vi "GUI_Single Button Pump.vi"() -> ()   [LabVIEW 2011] (continued)
            w1635 = T32[] [enum."Is BLT2 at Atmospheric Pressure?", enum."Is the EC Roughing Manifold at Atmospheric Pressure"] items=["No Action", "Is EC GPM Mode ON?", "Is EC GPM Mode Off?", "Is EC GVM Mode ON?", "Is EC GVM Off?", "Is  EC GPM or GVM Mode ON?", "Is LB GPM Mode ON?", "Is LB GPM Mode Off?", "Is LB GVM Mode ON?", "Is LB GVM Mode Off?", "Is  LB GPM or GVM Mode ON?", "Is M123 Turbo Gate Valve Opened? ", "Is M123 Turbo Gate Valve Closed?", "Is OAP Turbo Gate Valve Opened?", "Is OAP Turbo Gate Valve Closed?", "Is BTLTurbo Gate Valve Opened?", "Is BTL Turbo Gate Valve Closed?", "Is TARGET Turbo Gate Valve 1Opened?", "Is TARGET1 Turbo Gate Valve Closed?", "Is TARGET Turbo Gate Valve 2 Opened?", "Is TAREGT2 Turbo Gate Valve Closed?", "Is BTL2 Turbo Gate Valve Opened?", "Is BTL2 Turbo Gate Valve Closed?", "Is HPD Turbo Gate Valve Opened?", "Is HPD Turbo Gate Valve Closed?", "Is COMP to M123 gate Valve Opened?", "Is COMP to M123 Valve Closed?", "Is HPBD Gate Valve Opened?", "Is HPBD Gate Valve Closed?", "Is M123 to OAP gate valve opened?", "Is M123 to OAP gate valve closed?", "Is OAP to BLT gate valve opened?", "Is OAP to BTL Gate Valve Closed?", "Is BLT to TARGET gate valve opened?", "Is BTL to TARGET Gate Valve Closed?", "Is TARGET to BLT2 gate valve opened?", "Is TARGET to BTL2 Gate Valve Closed?", "Is BLT2 to HPD gate valve opened?", "Is BTL2 to HPD Gate Valve Closed?", "Is COMP at Atmospheric Pressure?", "Is M123 at Atmospheric Pressure?", "Is BeamDump at Atmospheric Pressure?", "Is OAP at Atmospheric Pressure?", "Is BLT at Atmospheric Pressure", "Is TARGET at Atmospheric Pressure?", "Is BLT2 at Atmospheric Pressure?", "Is HPD at Atmospheric Pressure?", "Is the EC Roughing Pump ON?", "Is the EC Roughing Pump OFF?", "Does the EC Roughing Pump have a fault?", "Is the LB Roughing Pump ON?", "Is the LB Roughing Pump Off?", "Does the LB Roughing Pump have a fault?", "Is the EC Backing Pump ON?", "Is the EC Backing Pump OFF?", "Is the LB Backing Pump ON?", "Is the LB Backing Pump OFF?", "Does the EC Backing Pump have a fault?", "Does the LB Backing Pump have a fault?", "Is the EC Backing Pipe at Atmospheric Pressure", "Is the LB Backing Pipe at Atmospheric Pressure", "Is the EC Backing Manifold at Atmospheric Pressure", "s the LB Backing Manifold at Atmospheric Pressure?", "Is the EC Roughing Pipe at Atmospheric Pressure", "Is the LB Roughing Pipe at Atmospheric Pressure?", "Is the EC Roughing Manifold at Atmospheric Pressure", "Is the LB Roughing Manifold at Atmospheric Pressure", "Is LB Backing Manifold Valve Opened?", "Is EC Backing Manifold Valve Opened?", "Is LB Roughing Manifold Valve Opened?", "Is EC Roughing Manifold Valve Opened?", "Is COMP Roughing Valve Opened?", "Is M123 Roughing Valve Opened?", "Is M123 Roughing Valve Closed?", "Is OAP Roughing Valve Opened?", "Is OAP Roughing Valve Closed?", "Is HPBD Roughing Valve Opened?", "Is HPBD Roughing Valve Closed?", "Is BTL Roughing Valve Opened?", "Is BTL Roughing Valve Closed?", "Is TARGET Roughing Valve Opened?", "Is TARGET Roughing Valve Closed?", "Is BTL2 Roughing Valve Opened?", "Is BTL2 Roughing Valve Closed?", "Is HPD Roughing Valve Opened?", "Is HPD Roughing Valve Closed?", "Is COMP Turbo Backing Valve Opened?", "Is M123 Turbo Backing Valve Opened", "Is HPBD Turbo Backing Valve Opened?", "Is OAP Turbo Backing Valve Opened?", "Is BTL Turbo Backing Valve Opened?", "Is TARGET1 Turbo Backing Valve Opened?", "Is TARGET2 Turbo Backing Valve Opened?", "Is BTL2 Turbo Backing Valve Opened?", "Is HPD Turbo Backing Valve Opened?", "Is M123 Backing at MID-VAC?", "Is OAP Backing at MID-VAC?", "Is TARGET1 Backing at MID-VAC?", "Is TARGET2 Backing at MID-VAC?", "Is BTL Backing at MID-VAC?", "Is BTL2 Backing at MID-VAC?", "Is HPD Backing at MID-VAC?", "Is M123 Turbo in Normal Operation", "Is COMP Turbo in Normal Operation", "Is OAP Turbo in Normal Operation", "Is BTL Turbo in Normal Operation", "Is TARGET1 Turbo in Normal Operation", "Is TARGET2 Turbo in Normal Operation", "Is BTL2 Turbo in Normal Operation", "Is HPD Turbo in Normal Operation", "Is M123 at MID-VAC?", "Is OAP at MID-VAC?", "Is COMP at MID-VAC?", "Is BTL at MID-VAC?", "Is TARGET at MID-VAC?", "Is BTL2 at MID-VAC?", "Is HPD at MID-VAC?"]
          }
          frame "HPD" {
            w1636 = T32[] [enum."Is HPD at Atmospheric Pressure?", enum."Is the EC Roughing Manifold at Atmospheric Pressure"] items=["No Action", "Is EC GPM Mode ON?", "Is EC GPM Mode Off?", "Is EC GVM Mode ON?", "Is EC GVM Off?", "Is  EC GPM or GVM Mode ON?", "Is LB GPM Mode ON?", "Is LB GPM Mode Off?", "Is LB GVM Mode ON?", "Is LB GVM Mode Off?", "Is  LB GPM or GVM Mode ON?", "Is M123 Turbo Gate Valve Opened? ", "Is M123 Turbo Gate Valve Closed?", "Is OAP Turbo Gate Valve Opened?", "Is OAP Turbo Gate Valve Closed?", "Is BTLTurbo Gate Valve Opened?", "Is BTL Turbo Gate Valve Closed?", "Is TARGET Turbo Gate Valve 1Opened?", "Is TARGET1 Turbo Gate Valve Closed?", "Is TARGET Turbo Gate Valve 2 Opened?", "Is TAREGT2 Turbo Gate Valve Closed?", "Is BTL2 Turbo Gate Valve Opened?", "Is BTL2 Turbo Gate Valve Closed?", "Is HPD Turbo Gate Valve Opened?", "Is HPD Turbo Gate Valve Closed?", "Is COMP to M123 gate Valve Opened?", "Is COMP to M123 Valve Closed?", "Is HPBD Gate Valve Opened?", "Is HPBD Gate Valve Closed?", "Is M123 to OAP gate valve opened?", "Is M123 to OAP gate valve closed?", "Is OAP to BLT gate valve opened?", "Is OAP to BTL Gate Valve Closed?", "Is BLT to TARGET gate valve opened?", "Is BTL to TARGET Gate Valve Closed?", "Is TARGET to BLT2 gate valve opened?", "Is TARGET to BTL2 Gate Valve Closed?", "Is BLT2 to HPD gate valve opened?", "Is BTL2 to HPD Gate Valve Closed?", "Is COMP at Atmospheric Pressure?", "Is M123 at Atmospheric Pressure?", "Is BeamDump at Atmospheric Pressure?", "Is OAP at Atmospheric Pressure?", "Is BLT at Atmospheric Pressure", "Is TARGET at Atmospheric Pressure?", "Is BLT2 at Atmospheric Pressure?", "Is HPD at Atmospheric Pressure?", "Is the EC Roughing Pump ON?", "Is the EC Roughing Pump OFF?", "Does the EC Roughing Pump have a fault?", "Is the LB Roughing Pump ON?", "Is the LB Roughing Pump Off?", "Does the LB Roughing Pump have a fault?", "Is the EC Backing Pump ON?", "Is the EC Backing Pump OFF?", "Is the LB Backing Pump ON?", "Is the LB Backing Pump OFF?", "Does the EC Backing Pump have a fault?", "Does the LB Backing Pump have a fault?", "Is the EC Backing Pipe at Atmospheric Pressure", "Is the LB Backing Pipe at Atmospheric Pressure", "Is the EC Backing Manifold at Atmospheric Pressure", "s the LB Backing Manifold at Atmospheric Pressure?", "Is the EC Roughing Pipe at Atmospheric Pressure", "Is the LB Roughing Pipe at Atmospheric Pressure?", "Is the EC Roughing Manifold at Atmospheric Pressure", "Is the LB Roughing Manifold at Atmospheric Pressure", "Is LB Backing Manifold Valve Opened?", "Is EC Backing Manifold Valve Opened?", "Is LB Roughing Manifold Valve Opened?", "Is EC Roughing Manifold Valve Opened?", "Is COMP Roughing Valve Opened?", "Is M123 Roughing Valve Opened?", "Is M123 Roughing Valve Closed?", "Is OAP Roughing Valve Opened?", "Is OAP Roughing Valve Closed?", "Is HPBD Roughing Valve Opened?", "Is HPBD Roughing Valve Closed?", "Is BTL Roughing Valve Opened?", "Is BTL Roughing Valve Closed?", "Is TARGET Roughing Valve Opened?", "Is TARGET Roughing Valve Closed?", "Is BTL2 Roughing Valve Opened?", "Is BTL2 Roughing Valve Closed?", "Is HPD Roughing Valve Opened?", "Is HPD Roughing Valve Closed?", "Is COMP Turbo Backing Valve Opened?", "Is M123 Turbo Backing Valve Opened", "Is HPBD Turbo Backing Valve Opened?", "Is OAP Turbo Backing Valve Opened?", "Is BTL Turbo Backing Valve Opened?", "Is TARGET1 Turbo Backing Valve Opened?", "Is TARGET2 Turbo Backing Valve Opened?", "Is BTL2 Turbo Backing Valve Opened?", "Is HPD Turbo Backing Valve Opened?", "Is M123 Backing at MID-VAC?", "Is OAP Backing at MID-VAC?", "Is TARGET1 Backing at MID-VAC?", "Is TARGET2 Backing at MID-VAC?", "Is BTL Backing at MID-VAC?", "Is BTL2 Backing at MID-VAC?", "Is HPD Backing at MID-VAC?", "Is M123 Turbo in Normal Operation", "Is COMP Turbo in Normal Operation", "Is OAP Turbo in Normal Operation", "Is BTL Turbo in Normal Operation", "Is TARGET1 Turbo in Normal Operation", "Is TARGET2 Turbo in Normal Operation", "Is BTL2 Turbo in Normal Operation", "Is HPD Turbo in Normal Operation", "Is M123 at MID-VAC?", "Is OAP at MID-VAC?", "Is COMP at MID-VAC?", "Is BTL at MID-VAC?", "Is TARGET at MID-VAC?", "Is BTL2 at MID-VAC?", "Is HPD at MID-VAC?"]
          }
        }
        n626 = call "GetAction.vi"("Check Condition"=w1606, "Query Array"=w1609, "input cluster"=w1600, "error in (no error)"=w1610) -> ("Status Array Out"=w1608:string[], "Generate Event?"=w1595:bool, "error out"=w1607:errorcluster)  [unwired: 6 in, 3 out]
        n627 = call "Generate User Event.vi"("Add(t)/Remove(f) Event"=w1595, "error in (no error)"=w1607, "User Event in"=w1612, "Status Array In"=w1608, "Error Codes"=w1606) -> ("error out"=w1611:errorcluster)  [unwired: 5 in, 1 out]
        n628 = case shown="\"M123\"" w1596 {
          tunnel: [w1615 "M123 chamber and the Roughing Manifold do not match in Pressure.\nPress Continue to Wait for 30 Seconds\nPress Exit to Quit" ("message") "HPBD Chamber and Roughing Manifold do not have matching Pressure.\nStop and Exit.(Restart the Pump down after all turbo valves have been manually closed)" ("message") "OAP Chamber and Roughing Manifold do not have matching Pressure.\nStop and Exit.(Restart the Pump down after all turbo valves have been manually closed)" ("message") "BTL Chamber and Roughing Manifold do not have matching Pressure.\nStop and Exit.(Restart the Pump down after all turbo valves have been manually closed)" ("message") "TARGET Chamber and Roughing Manifold do not have matching Pressure.\nStop and Exit.(Restart the Pump down after all turbo valves have been manually closed)" ("message") "BTL2 Chamber and Roughing Manifold do not have matching Pressure.\nStop and Exit.(Restart the Pump down after all turbo valves have been manually closed)" ("message") "HPD Chamber and Roughing Manifold do not have matching Pressure.\nStop and Exit.(Restart the Pump down after all turbo valves have been manually closed)" ("message")] -> w1602
          tunnel: [w1615 "Main: Roughing Valve Precheck>>M123" "Main: Roughing Valve Precheck>>HPBD" "Main: Roughing Valve Precheck>>OAP" "Main: Roughing Valve Precheck>>BTL" "Main: Roughing Valve Precheck>>TARGET" "Main: Roughing Valve Precheck>>BTL2" "Main: Roughing Valve Precheck>>HPD"] -> w1593
          frame "False", Default {
            w1615 = ""
          }
          frame "M123" {
          }
          frame "HPBD" {
          }
          frame "OAP" {
          }
          frame "BTL" {
          }
          frame "TARGET" {
          }
          frame "BTL2" {
          }
          frame "HPD" {
          }
        }
        n629 = call "MID-VAC Timer.vi"("Action"=timerAction_typdef."Timer Running") -> ("TO"=w1604:bool)  [unwired: 10 in]
        n630 = And(x=w1595, y=w1604) -> (x .and. y?=w1603:bool)
        n631 = Unbundle By Name(w1600) -> ("VI Refnum"=w1598:refnum<vi>)
        n632 = control-ref of="User Input Panel"() -> (w1599:refnum<vi>)
        n633 = call "Gen Next State based on user input.vi"("Next State IN"="", "Generate Event?"=w1595, "Idle State"=w1593, "Continue To Wait State"=w1593, "VI Refnum"=w1598, "SubPanel in"=w1599) -> ("Next State Out"=w1594:string)  [unwired: 5 in]
        n634 = call "Generate TO event.vi"("Boolean"=w1603, "message"=w1602, "User Event in"=w1601) -> ()  [unwired: 9 in]
        n635 = call <vilib>:"Add State(s) to Queue__jki_lib_state_machine.vi"("State(s) in Front (\"\")"=w1594, "State(s) in (\"\")"=w1614) -> ("States Out"=w1613:string)  [unwired: 13 in]
      }
      frame "Main: Open Roughing Valve" {
        # "Open Backing Valves on both systems"
        n636 = Unbundle By Name(w1641) -> ("TCPConnection.Command TCP Connection LB"=w1649:refnum<k5>)
        n637 = Unbundle By Name(w1641) -> ("TCPConnection.Command TCP Connection EC"=w1647:refnum<k5>)
        n638 = case shown="\"BTL2\"" w1639 {
          tunnel: [_ w1654 w1655 w1656 _ w1657 w1658 w1659 w1660] -> w1651
          frame "False", Default {
          }
          frame "M123" {
            w1654 = T33[] [enum."Open M123 Roughing Valve"] items=["No Action", "Set GPM Mode LB", "EXIT GPM Mode LB", "Set GPM Mode EC", "EXIT GPM Mode EC", "Set GVM mode LB", "Set GVM Mode EC", "Open LB Backing Valve", "Open EC Backing Valve", "Open EC Roughing Valve", "Open LB Roughing Valve", "Open M123 Roughing Valve", "Close M123 Roughing Valve", "Open Compressor Roughing Valve", "Close Compressor Roughing Valve", "Open BeamDump Roughing Valve", "Close BeamDump Roughing Valve", "Open OAP Roughing Valve", "Close OAP Roughing Valve", "Open BTL Roughing Valve", "Close BTL Roughing Valve", "Open Target Roughing Valve", "Close Target Roughing Valve", "Open BTL2 Roughing Valve", "Close BTL2 Roughing Valve", "Open HPD Roughing Valve", "Close HPD Roughing Valve", "LB Start Roughing Pump ", "EC Start Roughing Pump", "Open COMP Turbo Backing Valve", "Open M123 Turbo Backing Valve", "Open OAP Turbo Backing Valve", "Open HPBD Turbo Backing Valve", "Open BLT Turbo Backing Valve", "Open TARGET1 Turbo Backing Valve", "Open TARGET2 Turbo Backing Valve", "Open BLT2 Turbo Backing Valve", "Open HPD Turbo Backing Valve", "LB Start Turbo Backing Pump", "EC Start Turbo Backing Pump", "Start COMP Turbo Pump", "Start M123 Turbo Pump", "Start OAP Turbo Pump", "Start BTL Turbo Pump", "Start TARGET1 Turbo Pump", "Start TARGET2 Turbo Pump", "Start BTL2 Turbo Pump", "Start HPD Turbo Pump", "Open COMP Turbo Gate Valve", "Open M123 Turbo Gate Valve", "Open OAP Turbo Gate Valve", "Open BTL Turbo Gate Valve", "Open TARGET1 Turbo Gate Valve", "Open TARGET2 Turbo Gate Valve", "Open BTL2 Turbo Gate Valve", "Open HPD Turbo Gate Valve"]
          }
          frame "HPBD" {
            w1655 = T33[] [enum."Open BeamDump Roughing Valve"] items=["No Action", "Set GPM Mode LB", "EXIT GPM Mode LB", "Set GPM Mode EC", "EXIT GPM Mode EC", "Set GVM mode LB", "Set GVM Mode EC", "Open LB Backing Valve", "Open EC Backing Valve", "Open EC Roughing Valve", "Open LB Roughing Valve", "Open M123 Roughing Valve", "Close M123 Roughing Valve", "Open Compressor Roughing Valve", "Close Compressor Roughing Valve", "Open BeamDump Roughing Valve", "Close BeamDump Roughing Valve", "Open OAP Roughing Valve", "Close OAP Roughing Valve", "Open BTL Roughing Valve", "Close BTL Roughing Valve", "Open Target Roughing Valve", "Close Target Roughing Valve", "Open BTL2 Roughing Valve", "Close BTL2 Roughing Valve", "Open HPD Roughing Valve", "Close HPD Roughing Valve", "LB Start Roughing Pump ", "EC Start Roughing Pump", "Open COMP Turbo Backing Valve", "Open M123 Turbo Backing Valve", "Open OAP Turbo Backing Valve", "Open HPBD Turbo Backing Valve", "Open BLT Turbo Backing Valve", "Open TARGET1 Turbo Backing Valve", "Open TARGET2 Turbo Backing Valve", "Open BLT2 Turbo Backing Valve", "Open HPD Turbo Backing Valve", "LB Start Turbo Backing Pump", "EC Start Turbo Backing Pump", "Start COMP Turbo Pump", "Start M123 Turbo Pump", "Start OAP Turbo Pump", "Start BTL Turbo Pump", "Start TARGET1 Turbo Pump", "Start TARGET2 Turbo Pump", "Start BTL2 Turbo Pump", "Start HPD Turbo Pump", "Open COMP Turbo Gate Valve", "Open M123 Turbo Gate Valve", "Open OAP Turbo Gate Valve", "Open BTL Turbo Gate Valve", "Open TARGET1 Turbo Gate Valve", "Open TARGET2 Turbo Gate Valve", "Open BTL2 Turbo Gate Valve", "Open HPD Turbo Gate Valve"]
          }
          frame "OAP" {
            w1656 = T33[] [enum."Open OAP Roughing Valve"] items=["No Action", "Set GPM Mode LB", "EXIT GPM Mode LB", "Set GPM Mode EC", "EXIT GPM Mode EC", "Set GVM mode LB", "Set GVM Mode EC", "Open LB Backing Valve", "Open EC Backing Valve", "Open EC Roughing Valve", "Open LB Roughing Valve", "Open M123 Roughing Valve", "Close M123 Roughing Valve", "Open Compressor Roughing Valve", "Close Compressor Roughing Valve", "Open BeamDump Roughing Valve", "Close BeamDump Roughing Valve", "Open OAP Roughing Valve", "Close OAP Roughing Valve", "Open BTL Roughing Valve", "Close BTL Roughing Valve", "Open Target Roughing Valve", "Close Target Roughing Valve", "Open BTL2 Roughing Valve", "Close BTL2 Roughing Valve", "Open HPD Roughing Valve", "Close HPD Roughing Valve", "LB Start Roughing Pump ", "EC Start Roughing Pump", "Open COMP Turbo Backing Valve", "Open M123 Turbo Backing Valve", "Open OAP Turbo Backing Valve", "Open HPBD Turbo Backing Valve", "Open BLT Turbo Backing Valve", "Open TARGET1 Turbo Backing Valve", "Open TARGET2 Turbo Backing Valve", "Open BLT2 Turbo Backing Valve", "Open HPD Turbo Backing Valve", "LB Start Turbo Backing Pump", "EC Start Turbo Backing Pump", "Start COMP Turbo Pump", "Start M123 Turbo Pump", "Start OAP Turbo Pump", "Start BTL Turbo Pump", "Start TARGET1 Turbo Pump", "Start TARGET2 Turbo Pump", "Start BTL2 Turbo Pump", "Start HPD Turbo Pump", "Open COMP Turbo Gate Valve", "Open M123 Turbo Gate Valve", "Open OAP Turbo Gate Valve", "Open BTL Turbo Gate Valve", "Open TARGET1 Turbo Gate Valve", "Open TARGET2 Turbo Gate Valve", "Open BTL2 Turbo Gate Valve", "Open HPD Turbo Gate Valve"]
          }
          frame "COMP" {
          }
          frame "BTL" {
            w1657 = T33[] [enum."Open BTL Roughing Valve"] items=["No Action", "Set GPM Mode LB", "EXIT GPM Mode LB", "Set GPM Mode EC", "EXIT GPM Mode EC", "Set GVM mode LB", "Set GVM Mode EC", "Open LB Backing Valve", "Open EC Backing Valve", "Open EC Roughing Valve", "Open LB Roughing Valve", "Open M123 Roughing Valve", "Close M123 Roughing Valve", "Open Compressor Roughing Valve", "Close Compressor Roughing Valve", "Open BeamDump Roughing Valve", "Close BeamDump Roughing Valve", "Open OAP Roughing Valve", "Close OAP Roughing Valve", "Open BTL Roughing Valve", "Close BTL Roughing Valve", "Open Target Roughing Valve", "Close Target Roughing Valve", "Open BTL2 Roughing Valve", "Close BTL2 Roughing Valve", "Open HPD Roughing Valve", "Close HPD Roughing Valve", "LB Start Roughing Pump ", "EC Start Roughing Pump", "Open COMP Turbo Backing Valve", "Open M123 Turbo Backing Valve", "Open OAP Turbo Backing Valve", "Open HPBD Turbo Backing Valve", "Open BLT Turbo Backing Valve", "Open TARGET1 Turbo Backing Valve", "Open TARGET2 Turbo Backing Valve", "Open BLT2 Turbo Backing Valve", "Open HPD Turbo Backing Valve", "LB Start Turbo Backing Pump", "EC Start Turbo Backing Pump", "Start COMP Turbo Pump", "Start M123 Turbo Pump", "Start OAP Turbo Pump", "Start BTL Turbo Pump", "Start TARGET1 Turbo Pump", "Start TARGET2 Turbo Pump", "Start BTL2 Turbo Pump", "Start HPD Turbo Pump", "Open COMP Turbo Gate Valve", "Open M123 Turbo Gate Valve", "Open OAP Turbo Gate Valve", "Open BTL Turbo Gate Valve", "Open TARGET1 Turbo Gate Valve", "Open TARGET2 Turbo Gate Valve", "Open BTL2 Turbo Gate Valve", "Open HPD Turbo Gate Valve"]
          }
          frame "TARGET" {
            w1658 = T33[] [enum."Open Target Roughing Valve"] items=["No Action", "Set GPM Mode LB", "EXIT GPM Mode LB", "Set GPM Mode EC", "EXIT GPM Mode EC", "Set GVM mode LB", "Set GVM Mode EC", "Open LB Backing Valve", "Open EC Backing Valve", "Open EC Roughing Valve", "Open LB Roughing Valve", "Open M123 Roughing Valve", "Close M123 Roughing Valve", "Open Compressor Roughing Valve", "Close Compressor Roughing Valve", "Open BeamDump Roughing Valve", "Close BeamDump Roughing Valve", "Open OAP Roughing Valve", "Close OAP Roughing Valve", "Open BTL Roughing Valve", "Close BTL Roughing Valve", "Open Target Roughing Valve", "Close Target Roughing Valve", "Open BTL2 Roughing Valve", "Close BTL2 Roughing Valve", "Open HPD Roughing Valve", "Close HPD Roughing Valve", "LB Start Roughing Pump ", "EC Start Roughing Pump", "Open COMP Turbo Backing Valve", "Open M123 Turbo Backing Valve", "Open OAP Turbo Backing Valve", "Open HPBD Turbo Backing Valve", "Open BLT Turbo Backing Valve", "Open TARGET1 Turbo Backing Valve", "Open TARGET2 Turbo Backing Valve", "Open BLT2 Turbo Backing Valve", "Open HPD Turbo Backing Valve", "LB Start Turbo Backing Pump", "EC Start Turbo Backing Pump", "Start COMP Turbo Pump", "Start M123 Turbo Pump", "Start OAP Turbo Pump", "Start BTL Turbo Pump", "Start TARGET1 Turbo Pump", "Start TARGET2 Turbo Pump", "Start BTL2 Turbo Pump", "Start HPD Turbo Pump", "Open COMP Turbo Gate Valve", "Open M123 Turbo Gate Valve", "Open OAP Turbo Gate Valve", "Open BTL Turbo Gate Valve", "Open TARGET1 Turbo Gate Valve", "Open TARGET2 Turbo Gate Valve", "Open BTL2 Turbo Gate Valve", "Open HPD Turbo Gate Valve"]
          }
          frame "BTL2" {
            w1659 = T33[] [enum."Open BTL2 Roughing Valve"] items=["No Action", "Set GPM Mode LB", "EXIT GPM Mode LB", "Set GPM Mode EC", "EXIT GPM Mode EC", "Set GVM mode LB", "Set GVM Mode EC", "Open LB Backing Valve", "Open EC Backing Valve", "Open EC Roughing Valve", "Open LB Roughing Valve", "Open M123 Roughing Valve", "Close M123 Roughing Valve", "Open Compressor Roughing Valve", "Close Compressor Roughing Valve", "Open BeamDump Roughing Valve", "Close BeamDump Roughing Valve", "Open OAP Roughing Valve", "Close OAP Roughing Valve", "Open BTL Roughing Valve", "Close BTL Roughing Valve", "Open Target Roughing Valve", "Close Target Roughing Valve", "Open BTL2 Roughing Valve", "Close BTL2 Roughing Valve", "Open HPD Roughing Valve", "Close HPD Roughing Valve", "LB Start Roughing Pump ", "EC Start Roughing Pump", "Open COMP Turbo Backing Valve", "Open M123 Turbo Backing Valve", "Open OAP Turbo Backing Valve", "Open HPBD Turbo Backing Valve", "Open BLT Turbo Backing Valve", "Open TARGET1 Turbo Backing Valve", "Open TARGET2 Turbo Backing Valve", "Open BLT2 Turbo Backing Valve", "Open HPD Turbo Backing Valve", "LB Start Turbo Backing Pump", "EC Start Turbo Backing Pump", "Start COMP Turbo Pump", "Start M123 Turbo Pump", "Start OAP Turbo Pump", "Start BTL Turbo Pump", "Start TARGET1 Turbo Pump", "Start TARGET2 Turbo Pump", "Start BTL2 Turbo Pump", "Start HPD Turbo Pump", "Open COMP Turbo Gate Valve", "Open M123 Turbo Gate Valve", "Open OAP Turbo Gate Valve", "Open BTL Turbo Gate Valve", "Open TARGET1 Turbo Gate Valve", "Open TARGET2 Turbo Gate Valve", "Open BTL2 Turbo Gate Valve", "Open HPD Turbo Gate Valve"]
          }
          frame "HPD" {
            w1660 = T33[] [enum."Open HPD Roughing Valve"] items=["No Action", "Set GPM Mode LB", "EXIT GPM Mode LB", "Set GPM Mode EC", "EXIT GPM Mode EC", "Set GVM mode LB", "Set GVM Mode EC", "Open LB Backing Valve", "Open EC Backing Valve", "Open EC Roughing Valve", "Open LB Roughing Valve", "Open M123 Roughing Valve", "Close M123 Roughing Valve", "Open Compressor Roughing Valve", "Close Compressor Roughing Valve", "Open BeamDump Roughing Valve", "Close BeamDump Roughing Valve", "Open OAP Roughing Valve", "Close OAP Roughing Valve", "Open BTL Roughing Valve", "Close BTL Roughing Valve", "Open Target Roughing Valve", "Close Target Roughing Valve", "Open BTL2 Roughing Valve", "Close BTL2 Roughing Valve", "Open HPD Roughing Valve", "Close HPD Roughing Valve", "LB Start Roughing Pump ", "EC Start Roughing Pump", "Open COMP Turbo Backing Valve", "Open M123 Turbo Backing Valve", "Open OAP Turbo Backing Valve", "Open HPBD Turbo Backing Valve", "Open BLT Turbo Backing Valve", "Open TARGET1 Turbo Backing Valve", "Open TARGET2 Turbo Backing Valve", "Open BLT2 Turbo Backing Valve", "Open HPD Turbo Backing Valve", "LB Start Turbo Backing Pump", "EC Start Turbo Backing Pump", "Start COMP Turbo Pump", "Start M123 Turbo Pump", "Start OAP Turbo Pump", "Start BTL Turbo Pump", "Start TARGET1 Turbo Pump", "Start TARGET2 Turbo Pump", "Start BTL2 Turbo Pump", "Start HPD Turbo Pump", "Open COMP Turbo Gate Valve", "Open M123 Turbo Gate Valve", "Open OAP Turbo Gate Valve", "Open BTL Turbo Gate Valve", "Open TARGET1 Turbo Gate Valve", "Open TARGET2 Turbo Gate Valve", "Open BTL2 Turbo Gate Valve", "Open HPD Turbo Gate Valve"]
          }
        }
        n639 = call "Build Command.vi"("Command Array in"=w1651, "input cluster"=w1641) -> ("output EC Command cluster"=w1648:T34, "output LB Command cluster"=w1650:T34)  [unwired: 8 in]
        n640 = call "Send Command LB.vi"("error in (no error)"=w1646, "output LB Command cluster"=w1650, "TCP Network Connection in"=w1649) -> ("error out"=w1644:errorcluster)  [unwired: 8 in]
        n641 = call "Send Command EC.vi"("error in (no error)"=w1646, "output EC Command cluster"=w1648, "TCP Network Connection in"=w1647) -> ("error out"=w1645:errorcluster)  [unwired: 8 in]
        n642 = Merge Errors(w1644, w1645) -> (w1643:errorcluster)
        n643 = call "Reset Command Clusters.vi"("error in (no error)"=w1643, "input cluster"=w1641) -> ("error out"=w1642:errorcluster, "output cluster"=w1640:T20)  [unwired: 8 in]
        n644 = call "MID-VAC Timer.vi"("TO sec (Start timer)"=5.0, "Action"=timerAction_typdef."Start Timer") -> ()  [unwired: 9 in, 1 out]
        n645 = call <vilib>:"Add State(s) to Queue__jki_lib_state_machine.vi"("State(s) in (\"\")"=w1653) -> ("States Out"=w1652:string)  [unwired: 14 in]
      }
      frame "Main: Check Roughing Valve Status" {
        w1678 = Error_codes."010-Roughing Valve Status" ("Error Codes")
        # "Event TAG"
        n646 = case shown="\"M123\"" w1673 {
          tunnel: [_ w1699 w1700 w1701 _ w1702 _ _ w1703] -> w1674
          frame "False", Default {
          }
          frame "M123" {
            w1699 = T32[] [enum."Is M123 Roughing Valve Opened?"] items=["No Action", "Is EC GPM Mode ON?", "Is EC GPM Mode Off?", "Is EC GVM Mode ON?", "Is EC GVM Off?", "Is  EC GPM or GVM Mode ON?", "Is LB GPM Mode ON?", "Is LB GPM Mode Off?", "Is LB GVM Mode ON?", "Is LB GVM Mode Off?", "Is  LB GPM or GVM Mode ON?", "Is M123 Turbo Gate Valve Opened? ", "Is M123 Turbo Gate Valve Closed?", "Is OAP Turbo Gate Valve Opened?", "Is OAP Turbo Gate Valve Closed?", "Is BTLTurbo Gate Valve Opened?", "Is BTL Turbo Gate Valve Closed?", "Is TARGET Turbo Gate Valve 1Opened?", "Is TARGET1 Turbo Gate Valve Closed?", "Is TARGET Turbo Gate Valve 2 Opened?", "Is TAREGT2 Turbo Gate Valve Closed?", "Is BTL2 Turbo Gate Valve Opened?", "Is BTL2 Turbo Gate Valve Closed?", "Is HPD Turbo Gate Valve Opened?", "Is HPD Turbo Gate Valve Closed?", "Is COMP to M123 gate Valve Opened?", "Is COMP to M123 Valve Closed?", "Is HPBD Gate Valve Opened?", "Is HPBD Gate Valve Closed?", "Is M123 to OAP gate valve opened?", "Is M123 to OAP gate valve closed?", "Is OAP to BLT gate valve opened?", "Is OAP to BTL Gate Valve Closed?", "Is BLT to TARGET gate valve opened?", "Is BTL to TARGET Gate Valve Closed?", "Is TARGET to BLT2 gate valve opened?", "Is TARGET to BTL2 Gate Valve Closed?", "Is BLT2 to HPD gate valve opened?", "Is BTL2 to HPD Gate Valve Closed?", "Is COMP at Atmospheric Pressure?", "Is M123 at Atmospheric Pressure?", "Is BeamDump at Atmospheric Pressure?", "Is OAP at Atmospheric Pressure?", "Is BLT at Atmospheric Pressure", "Is TARGET at Atmospheric Pressure?", "Is BLT2 at Atmospheric Pressure?", "Is HPD at Atmospheric Pressure?", "Is the EC Roughing Pump ON?", "Is the EC Roughing Pump OFF?", "Does the EC Roughing Pump have a fault?", "Is the LB Roughing Pump ON?", "Is the LB Roughing Pump Off?", "Does the LB Roughing Pump have a fault?", "Is the EC Backing Pump ON?", "Is the EC Backing Pump OFF?", "Is the LB Backing Pump ON?", "Is the LB Backing Pump OFF?", "Does the EC Backing Pump have a fault?", "Does the LB Backing Pump have a fault?", "Is the EC Backing Pipe at Atmospheric Pressure", "Is the LB Backing Pipe at Atmospheric Pressure", "Is the EC Backing Manifold at Atmospheric Pressure", "s the LB Backing Manifold at Atmospheric Pressure?", "Is the EC Roughing Pipe at Atmospheric Pressure", "Is the LB Roughing Pipe at Atmospheric Pressure?", "Is the EC Roughing Manifold at Atmospheric Pressure", "Is the LB Roughing Manifold at Atmospheric Pressure", "Is LB Backing Manifold Valve Opened?", "Is EC Backing Manifold Valve Opened?", "Is LB Roughing Manifold Valve Opened?", "Is EC Roughing Manifold Valve Opened?", "Is COMP Roughing Valve Opened?", "Is M123 Roughing Valve Opened?", "Is M123 Roughing Valve Closed?", "Is OAP Roughing Valve Opened?", "Is OAP Roughing Valve Closed?", "Is HPBD Roughing Valve Opened?", "Is HPBD Roughing Valve Closed?", "Is BTL Roughing Valve Opened?", "Is BTL Roughing Valve Closed?", "Is TARGET Roughing Valve Opened?", "Is TARGET Roughing Valve Closed?", "Is BTL2 Roughing Valve Opened?", "Is BTL2 Roughing Valve Closed?", "Is HPD Roughing Valve Opened?", "Is HPD Roughing Valve Closed?", "Is COMP Turbo Backing Valve Opened?", "Is M123 Turbo Backing Valve Opened", "Is HPBD Turbo Backing Valve Opened?", "Is OAP Turbo Backing Valve Opened?", "Is BTL Turbo Backing Valve Opened?", "Is TARGET1 Turbo Backing Valve Opened?", "Is TARGET2 Turbo Backing Valve Opened?", "Is BTL2 Turbo Backing Valve Opened?", "Is HPD Turbo Backing Valve Opened?", "Is M123 Backing at MID-VAC?", "Is OAP Backing at MID-VAC?", "Is TARGET1 Backing at MID-VAC?", "Is TARGET2 Backing at MID-VAC?", "Is BTL Backing at MID-VAC?", "Is BTL2 Backing at MID-VAC?", "Is HPD Backing at MID-VAC?", "Is M123 Turbo in Normal Operation", "Is COMP Turbo in Normal Operation", "Is OAP Turbo in Normal Operation", "Is BTL Turbo in Normal Operation", "Is TARGET1 Turbo in Normal Operation", "Is TARGET2 Turbo in Normal Operation", "Is BTL2 Turbo in Normal Operation", "Is HPD Turbo in Normal Operation", "Is M123 at MID-VAC?", "Is OAP at MID-VAC?", "Is COMP at MID-VAC?", "Is BTL at MID-VAC?", "Is TARGET at MID-VAC?", "Is BTL2 at MID-VAC?", "Is HPD at MID-VAC?"]
          }
          frame "HPBD" {
            w1700 = T32[] [enum."Is HPBD Roughing Valve Opened?"] items=["No Action", "Is EC GPM Mode ON?", "Is EC GPM Mode Off?", "Is EC GVM Mode ON?", "Is EC GVM Off?", "Is  EC GPM or GVM Mode ON?", "Is LB GPM Mode ON?", "Is LB GPM Mode Off?", "Is LB GVM Mode ON?", "Is LB GVM Mode Off?", "Is  LB GPM or GVM Mode ON?", "Is M123 Turbo Gate Valve Opened? ", "Is M123 Turbo Gate Valve Closed?", "Is OAP Turbo Gate Valve Opened?", "Is OAP Turbo Gate Valve Closed?", "Is BTLTurbo Gate Valve Opened?", "Is BTL Turbo Gate Valve Closed?", "Is TARGET Turbo Gate Valve 1Opened?", "Is TARGET1 Turbo Gate Valve Closed?", "Is TARGET Turbo Gate Valve 2 Opened?", "Is TAREGT2 Turbo Gate Valve Closed?", "Is BTL2 Turbo Gate Valve Opened?", "Is BTL2 Turbo Gate Valve Closed?", "Is HPD Turbo Gate Valve Opened?", "Is HPD Turbo Gate Valve Closed?", "Is COMP to M123 gate Valve Opened?", "Is COMP to M123 Valve Closed?", "Is HPBD Gate Valve Opened?", "Is HPBD Gate Valve Closed?", "Is M123 to OAP gate valve opened?", "Is M123 to OAP gate valve closed?", "Is OAP to BLT gate valve opened?", "Is OAP to BTL Gate Valve Closed?", "Is BLT to TARGET gate valve opened?", "Is BTL to TARGET Gate Valve Closed?", "Is TARGET to BLT2 gate valve opened?", "Is TARGET to BTL2 Gate Valve Closed?", "Is BLT2 to HPD gate valve opened?", "Is BTL2 to HPD Gate Valve Closed?", "Is COMP at Atmospheric Pressure?", "Is M123 at Atmospheric Pressure?", "Is BeamDump at Atmospheric Pressure?", "Is OAP at Atmospheric Pressure?", "Is BLT at Atmospheric Pressure", "Is TARGET at Atmospheric Pressure?", "Is BLT2 at Atmospheric Pressure?", "Is HPD at Atmospheric Pressure?", "Is the EC Roughing Pump ON?", "Is the EC Roughing Pump OFF?", "Does the EC Roughing Pump have a fault?", "Is the LB Roughing Pump ON?", "Is the LB Roughing Pump Off?", "Does the LB Roughing Pump have a fault?", "Is the EC Backing Pump ON?", "Is the EC Backing Pump OFF?", "Is the LB Backing Pump ON?", "Is the LB Backing Pump OFF?", "Does the EC Backing Pump have a fault?", "Does the LB Backing Pump have a fault?", "Is the EC Backing Pipe at Atmospheric Pressure", "Is the LB Backing Pipe at Atmospheric Pressure", "Is the EC Backing Manifold at Atmospheric Pressure", "s the LB Backing Manifold at Atmospheric Pressure?", "Is the EC Roughing Pipe at Atmospheric Pressure", "Is the LB Roughing Pipe at Atmospheric Pressure?", "Is the EC Roughing Manifold at Atmospheric Pressure", "Is the LB Roughing Manifold at Atmospheric Pressure", "Is LB Backing Manifold Valve Opened?", "Is EC Backing Manifold Valve Opened?", "Is LB Roughing Manifold Valve Opened?", "Is EC Roughing Manifold Valve Opened?", "Is COMP Roughing Valve Opened?", "Is M123 Roughing Valve Opened?", "Is M123 Roughing Valve Closed?", "Is OAP Roughing Valve Opened?", "Is OAP Roughing Valve Closed?", "Is HPBD Roughing Valve Opened?", "Is HPBD Roughing Valve Closed?", "Is BTL Roughing Valve Opened?", "Is BTL Roughing Valve Closed?", "Is TARGET Roughing Valve Opened?", "Is TARGET Roughing Valve Closed?", "Is BTL2 Roughing Valve Opened?", "Is BTL2 Roughing Valve Closed?", "Is HPD Roughing Valve Opened?", "Is HPD Roughing Valve Closed?", "Is COMP Turbo Backing Valve Opened?", "Is M123 Turbo Backing Valve Opened", "Is HPBD Turbo Backing Valve Opened?", "Is OAP Turbo Backing Valve Opened?", "Is BTL Turbo Backing Valve Opened?", "Is TARGET1 Turbo Backing Valve Opened?", "Is TARGET2 Turbo Backing Valve Opened?", "Is BTL2 Turbo Backing Valve Opened?", "Is HPD Turbo Backing Valve Opened?", "Is M123 Backing at MID-VAC?", "Is OAP Backing at MID-VAC?", "Is TARGET1 Backing at MID-VAC?", "Is TARGET2 Backing at MID-VAC?", "Is BTL Backing at MID-VAC?", "Is BTL2 Backing at MID-VAC?", "Is HPD Backing at MID-VAC?", "Is M123 Turbo in Normal Operation", "Is COMP Turbo in Normal Operation", "Is OAP Turbo in Normal Operation", "Is BTL Turbo in Normal Operation", "Is TARGET1 Turbo in Normal Operation", "Is TARGET2 Turbo in Normal Operation", "Is BTL2 Turbo in Normal Operation", "Is HPD Turbo in Normal Operation", "Is M123 at MID-VAC?", "Is OAP at MID-VAC?", "Is COMP at MID-VAC?", "Is BTL at MID-VAC?", "Is TARGET at MID-VAC?", "Is BTL2 at MID-VAC?", "Is HPD at MID-VAC?"]
          }
          frame "OAP" {
            w1701 = T32[] [enum."Is OAP Roughing Valve Opened?"] items=["No Action", "Is EC GPM Mode ON?", "Is EC GPM Mode Off?", "Is EC GVM Mode ON?", "Is EC GVM Off?", "Is  EC GPM or GVM Mode ON?", "Is LB GPM Mode ON?", "Is LB GPM Mode Off?", "Is LB GVM Mode ON?", "Is LB GVM Mode Off?", "Is  LB GPM or GVM Mode ON?", "Is M123 Turbo Gate Valve Opened? ", "Is M123 Turbo Gate Valve Closed?", "Is OAP Turbo Gate Valve Opened?", "Is OAP Turbo Gate Valve Closed?", "Is BTLTurbo Gate Valve Opened?", "Is BTL Turbo Gate Valve Closed?", "Is TARGET Turbo Gate Valve 1Opened?", "Is TARGET1 Turbo Gate Valve Closed?", "Is TARGET Turbo Gate Valve 2 Opened?", "Is TAREGT2 Turbo Gate Valve Closed?", "Is BTL2 Turbo Gate Valve Opened?", "Is BTL2 Turbo Gate Valve Closed?", "Is HPD Turbo Gate Valve Opened?", "Is HPD Turbo Gate Valve Closed?", "Is COMP to M123 gate Valve Opened?", "Is COMP to M123 Valve Closed?", "Is HPBD Gate Valve Opened?", "Is HPBD Gate Valve Closed?", "Is M123 to OAP gate valve opened?", "Is M123 to OAP gate valve closed?", "Is OAP to BLT gate valve opened?", "Is OAP to BTL Gate Valve Closed?", "Is BLT to TARGET gate valve opened?", "Is BTL to TARGET Gate Valve Closed?", "Is TARGET to BLT2 gate valve opened?", "Is TARGET to BTL2 Gate Valve Closed?", "Is BLT2 to HPD gate valve opened?", "Is BTL2 to HPD Gate Valve Closed?", "Is COMP at Atmospheric Pressure?", "Is M123 at Atmospheric Pressure?", "Is BeamDump at Atmospheric Pressure?", "Is OAP at Atmospheric Pressure?", "Is BLT at Atmospheric Pressure", "Is TARGET at Atmospheric Pressure?", "Is BLT2 at Atmospheric Pressure?", "Is HPD at Atmospheric Pressure?", "Is the EC Roughing Pump ON?", "Is the EC Roughing Pump OFF?", "Does the EC Roughing Pump have a fault?", "Is the LB Roughing Pump ON?", "Is the LB Roughing Pump Off?", "Does the LB Roughing Pump have a fault?", "Is the EC Backing Pump ON?", "Is the EC Backing Pump OFF?", "Is the LB Backing Pump ON?", "Is the LB Backing Pump OFF?", "Does the EC Backing Pump have a fault?", "Does the LB Backing Pump have a fault?", "Is the EC Backing Pipe at Atmospheric Pressure", "Is the LB Backing Pipe at Atmospheric Pressure", "Is the EC Backing Manifold at Atmospheric Pressure", "s the LB Backing Manifold at Atmospheric Pressure?", "Is the EC Roughing Pipe at Atmospheric Pressure", "Is the LB Roughing Pipe at Atmospheric Pressure?", "Is the EC Roughing Manifold at Atmospheric Pressure", "Is the LB Roughing Manifold at Atmospheric Pressure", "Is LB Backing Manifold Valve Opened?", "Is EC Backing Manifold Valve Opened?", "Is LB Roughing Manifold Valve Opened?", "Is EC Roughing Manifold Valve Opened?", "Is COMP Roughing Valve Opened?", "Is M123 Roughing Valve Opened?", "Is M123 Roughing Valve Closed?", "Is OAP Roughing Valve Opened?", "Is OAP Roughing Valve Closed?", "Is HPBD Roughing Valve Opened?", "Is HPBD Roughing Valve Closed?", "Is BTL Roughing Valve Opened?", "Is BTL Roughing Valve Closed?", "Is TARGET Roughing Valve Opened?", "Is TARGET Roughing Valve Closed?", "Is BTL2 Roughing Valve Opened?", "Is BTL2 Roughing Valve Closed?", "Is HPD Roughing Valve Opened?", "Is HPD Roughing Valve Closed?", "Is COMP Turbo Backing Valve Opened?", "Is M123 Turbo Backing Valve Opened", "Is HPBD Turbo Backing Valve Opened?", "Is OAP Turbo Backing Valve Opened?", "Is BTL Turbo Backing Valve Opened?", "Is TARGET1 Turbo Backing Valve Opened?", "Is TARGET2 Turbo Backing Valve Opened?", "Is BTL2 Turbo Backing Valve Opened?", "Is HPD Turbo Backing Valve Opened?", "Is M123 Backing at MID-VAC?", "Is OAP Backing at MID-VAC?", "Is TARGET1 Backing at MID-VAC?", "Is TARGET2 Backing at MID-VAC?", "Is BTL Backing at MID-VAC?", "Is BTL2 Backing at MID-VAC?", "Is HPD Backing at MID-VAC?", "Is M123 Turbo in Normal Operation", "Is COMP Turbo in Normal Operation", "Is OAP Turbo in Normal Operation", "Is BTL Turbo in Normal Operation", "Is TARGET1 Turbo in Normal Operation", "Is TARGET2 Turbo in Normal Operation", "Is BTL2 Turbo in Normal Operation", "Is HPD Turbo in Normal Operation", "Is M123 at MID-VAC?", "Is OAP at MID-VAC?", "Is COMP at MID-VAC?", "Is BTL at MID-VAC?", "Is TARGET at MID-VAC?", "Is BTL2 at MID-VAC?", "Is HPD at MID-VAC?"]
          }
          frame "COMP" {
          }
          frame "BTL" {
            w1702 = T32[] [enum."Is BTL Roughing Valve Opened?"] items=["No Action", "Is EC GPM Mode ON?", "Is EC GPM Mode Off?", "Is EC GVM Mode ON?", "Is EC GVM Off?", "Is  EC GPM or GVM Mode ON?", "Is LB GPM Mode ON?", "Is LB GPM Mode Off?", "Is LB GVM Mode ON?", "Is LB GVM Mode Off?", "Is  LB GPM or GVM Mode ON?", "Is M123 Turbo Gate Valve Opened? ", "Is M123 Turbo Gate Valve Closed?", "Is OAP Turbo Gate Valve Opened?", "Is OAP Turbo Gate Valve Closed?", "Is BTLTurbo Gate Valve Opened?", "Is BTL Turbo Gate Valve Closed?", "Is TARGET Turbo Gate Valve 1Opened?", "Is TARGET1 Turbo Gate Valve Closed?", "Is TARGET Turbo Gate Valve 2 Opened?", "Is TAREGT2 Turbo Gate Valve Closed?", "Is BTL2 Turbo Gate Valve Opened?", "Is BTL2 Turbo Gate Valve Closed?", "Is HPD Turbo Gate Valve Opened?", "Is HPD Turbo Gate Valve Closed?", "Is COMP to M123 gate Valve Opened?", "Is COMP to M123 Valve Closed?", "Is HPBD Gate Valve Opened?", "Is HPBD Gate Valve Closed?", "Is M123 to OAP gate valve opened?", "Is M123 to OAP gate valve closed?", "Is OAP to BLT gate valve opened?", "Is OAP to BTL Gate Valve Closed?", "Is BLT to TARGET gate valve opened?", "Is BTL to TARGET Gate Valve Closed?", "Is TARGET to BLT2 gate valve opened?", "Is TARGET to BTL2 Gate Valve Closed?", "Is BLT2 to HPD gate valve opened?", "Is BTL2 to HPD Gate Valve Closed?", "Is COMP at Atmospheric Pressure?", "Is M123 at Atmospheric Pressure?", "Is BeamDump at Atmospheric Pressure?", "Is OAP at Atmospheric Pressure?", "Is BLT at Atmospheric Pressure", "Is TARGET at Atmospheric Pressure?", "Is BLT2 at Atmospheric Pressure?", "Is HPD at Atmospheric Pressure?", "Is the EC Roughing Pump ON?", "Is the EC Roughing Pump OFF?", "Does the EC Roughing Pump have a fault?", "Is the LB Roughing Pump ON?", "Is the LB Roughing Pump Off?", "Does the LB Roughing Pump have a fault?", "Is the EC Backing Pump ON?", "Is the EC Backing Pump OFF?", "Is the LB Backing Pump ON?", "Is the LB Backing Pump OFF?", "Does the EC Backing Pump have a fault?", "Does the LB Backing Pump have a fault?", "Is the EC Backing Pipe at Atmospheric Pressure", "Is the LB Backing Pipe at Atmospheric Pressure", "Is the EC Backing Manifold at Atmospheric Pressure", "s the LB Backing Manifold at Atmospheric Pressure?", "Is the EC Roughing Pipe at Atmospheric Pressure", "Is the LB Roughing Pipe at Atmospheric Pressure?", "Is the EC Roughing Manifold at Atmospheric Pressure", "Is the LB Roughing Manifold at Atmospheric Pressure", "Is LB Backing Manifold Valve Opened?", "Is EC Backing Manifold Valve Opened?", "Is LB Roughing Manifold Valve Opened?", "Is EC Roughing Manifold Valve Opened?", "Is COMP Roughing Valve Opened?", "Is M123 Roughing Valve Opened?", "Is M123 Roughing Valve Closed?", "Is OAP Roughing Valve Opened?", "Is OAP Roughing Valve Closed?", "Is HPBD Roughing Valve Opened?", "Is HPBD Roughing Valve Closed?", "Is BTL Roughing Valve Opened?", "Is BTL Roughing Valve Closed?", "Is TARGET Roughing Valve Opened?", "Is TARGET Roughing Valve Closed?", "Is BTL2 Roughing Valve Opened?", "Is BTL2 Roughing Valve Closed?", "Is HPD Roughing Valve Opened?", "Is HPD Roughing Valve Closed?", "Is COMP Turbo Backing Valve Opened?", "Is M123 Turbo Backing Valve Opened", "Is HPBD Turbo Backing Valve Opened?", "Is OAP Turbo Backing Valve Opened?", "Is BTL Turbo Backing Valve Opened?", "Is TARGET1 Turbo Backing Valve Opened?", "Is TARGET2 Turbo Backing Valve Opened?", "Is BTL2 Turbo Backing Valve Opened?", "Is HPD Turbo Backing Valve Opened?", "Is M123 Backing at MID-VAC?", "Is OAP Backing at MID-VAC?", "Is TARGET1 Backing at MID-VAC?", "Is TARGET2 Backing at MID-VAC?", "Is BTL Backing at MID-VAC?", "Is BTL2 Backing at MID-VAC?", "Is HPD Backing at MID-VAC?", "Is M123 Turbo in Normal Operation", "Is COMP Turbo in Normal Operation", "Is OAP Turbo in Normal Operation", "Is BTL Turbo in Normal Operation", "Is TARGET1 Turbo in Normal Operation", "Is TARGET2 Turbo in Normal Operation", "Is BTL2 Turbo in Normal Operation", "Is HPD Turbo in Normal Operation", "Is M123 at MID-VAC?", "Is OAP at MID-VAC?", "Is COMP at MID-VAC?", "Is BTL at MID-VAC?", "Is TARGET at MID-VAC?", "Is BTL2 at MID-VAC?", "Is HPD at MID-VAC?"]
          }
          frame "TARGET" {
            (unwired) T32[] [enum."Is TARGET Roughing Valve Opened?"] items=["No Action", "Is EC GPM Mode ON?", "Is EC GPM Mode Off?", "Is EC GVM Mode ON?", "Is EC GVM Off?", "Is  EC GPM or GVM Mode ON?", "Is LB GPM Mode ON?", "Is LB GPM Mode Off?", "Is LB GVM Mode ON?", "Is LB GVM Mode Off?", "Is  LB GPM or GVM Mode ON?", "Is M123 Turbo Gate Valve Opened? ", "Is M123 Turbo Gate Valve Closed?", "Is OAP Turbo Gate Valve Opened?", "Is OAP Turbo Gate Valve Closed?", "Is BTLTurbo Gate Valve Opened?", "Is BTL Turbo Gate Valve Closed?", "Is TARGET Turbo Gate Valve 1Opened?", "Is TARGET1 Turbo Gate Valve Closed?", "Is TARGET Turbo Gate Valve 2 Opened?", "Is TAREGT2 Turbo Gate Valve Closed?", "Is BTL2 Turbo Gate Valve Opened?", "Is BTL2 Turbo Gate Valve Closed?", "Is HPD Turbo Gate Valve Opened?", "Is HPD Turbo Gate Valve Closed?", "Is COMP to M123 gate Valve Opened?", "Is COMP to M123 Valve Closed?", "Is HPBD Gate Valve Opened?", "Is HPBD Gate Valve Closed?", "Is M123 to OAP gate valve opened?", "Is M123 to OAP gate valve closed?", "Is OAP to BLT gate valve opened?", "Is OAP to BTL Gate Valve Closed?", "Is BLT to TARGET gate valve opened?", "Is BTL to TARGET Gate Valve Closed?", "Is TARGET to BLT2 gate valve opened?", "Is TARGET to BTL2 Gate Valve Closed?", "Is BLT2 to HPD gate valve opened?", "Is BTL2 to HPD Gate Valve Closed?", "Is COMP at Atmospheric Pressure?", "Is M123 at Atmospheric Pressure?", "Is BeamDump at Atmospheric Pressure?", "Is OAP at Atmospheric Pressure?", "Is BLT at Atmospheric Pressure", "Is TARGET at Atmospheric Pressure?", "Is BLT2 at Atmospheric Pressure?", "Is HPD at Atmospheric Pressure?", "Is the EC Roughing Pump ON?", "Is the EC Roughing Pump OFF?", "Does the EC Roughing Pump have a fault?", "Is the LB Roughing Pump ON?", "Is the LB Roughing Pump Off?", "Does the LB Roughing Pump have a fault?", "Is the EC Backing Pump ON?", "Is the EC Backing Pump OFF?", "Is the LB Backing Pump ON?", "Is the LB Backing Pump OFF?", "Does the EC Backing Pump have a fault?", "Does the LB Backing Pump have a fault?", "Is the EC Backing Pipe at Atmospheric Pressure", "Is the LB Backing Pipe at Atmospheric Pressure", "Is the EC Backing Manifold at Atmospheric Pressure", "s the LB Backing Manifold at Atmospheric Pressure?", "Is the EC Roughing Pipe at Atmospheric Pressure", "Is the LB Roughing Pipe at Atmospheric Pressure?", "Is the EC Roughing Manifold at Atmospheric Pressure", "Is the LB Roughing Manifold at Atmospheric Pressure", "Is LB Backing Manifold Valve Opened?", "Is EC Backing Manifold Valve Opened?", "Is LB Roughing Manifold Valve Opened?", "Is EC Roughing Manifold Valve Opened?", "Is COMP Roughing Valve Opened?", "Is M123 Roughing Valve Opened?", "Is M123 Roughing Valve Closed?", "Is OAP Roughing Valve Opened?", "Is OAP Roughing Valve Closed?", "Is HPBD Roughing Valve Opened?", "Is HPBD Roughing Valve Closed?", "Is BTL Roughing Valve Opened?", "Is BTL Roughing Valve Closed?", "Is TARGET Roughing Valve Opened?", "Is TARGET Roughing Valve Closed?", "Is BTL2 Roughing Valve Opened?", "Is BTL2 Roughing Valve Closed?", "Is HPD Roughing Valve Opened?", "Is HPD Roughing Valve Closed?", "Is COMP Turbo Backing Valve Opened?", "Is M123 Turbo Backing Valve Opened", "Is HPBD Turbo Backing Valve Opened?", "Is OAP Turbo Backing Valve Opened?", "Is BTL Turbo Backing Valve Opened?", "Is TARGET1 Turbo Backing Valve Opened?", "Is TARGET2 Turbo Backing Valve Opened?", "Is BTL2 Turbo Backing Valve Opened?", "Is HPD Turbo Backing Valve Opened?", "Is M123 Backing at MID-VAC?", "Is OAP Backing at MID-VAC?", "Is TARGET1 Backing at MID-VAC?", "Is TARGET2 Backing at MID-VAC?", "Is BTL Backing at MID-VAC?", "Is BTL2 Backing at MID-VAC?", "Is HPD Backing at MID-VAC?", "Is M123 Turbo in Normal Operation", "Is COMP Turbo in Normal Operation", "Is OAP Turbo in Normal Operation", "Is BTL Turbo in Normal Operation", "Is TARGET1 Turbo in Normal Operation", "Is TARGET2 Turbo in Normal Operation", "Is BTL2 Turbo in Normal Operation", "Is HPD Turbo in Normal Operation", "Is M123 at MID-VAC?", "Is OAP at MID-VAC?", "Is COMP at MID-VAC?", "Is BTL at MID-VAC?", "Is TARGET at MID-VAC?", "Is BTL2 at MID-VAC?", "Is HPD at MID-VAC?"]
          }
          frame "BTL2" {
            (unwired) T32[] [enum."Is BTL2 Roughing Valve Opened?"] items=["No Action", "Is EC GPM Mode ON?", "Is EC GPM Mode Off?", "Is EC GVM Mode ON?", "Is EC GVM Off?", "Is  EC GPM or GVM Mode ON?", "Is LB GPM Mode ON?", "Is LB GPM Mode Off?", "Is LB GVM Mode ON?", "Is LB GVM Mode Off?", "Is  LB GPM or GVM Mode ON?", "Is M123 Turbo Gate Valve Opened? ", "Is M123 Turbo Gate Valve Closed?", "Is OAP Turbo Gate Valve Opened?", "Is OAP Turbo Gate Valve Closed?", "Is BTLTurbo Gate Valve Opened?", "Is BTL Turbo Gate Valve Closed?", "Is TARGET Turbo Gate Valve 1Opened?", "Is TARGET1 Turbo Gate Valve Closed?", "Is TARGET Turbo Gate Valve 2 Opened?", "Is TAREGT2 Turbo Gate Valve Closed?", "Is BTL2 Turbo Gate Valve Opened?", "Is BTL2 Turbo Gate Valve Closed?", "Is HPD Turbo Gate Valve Opened?", "Is HPD Turbo Gate Valve Closed?", "Is COMP to M123 gate Valve Opened?", "Is COMP to M123 Valve Closed?", "Is HPBD Gate Valve Opened?", "Is HPBD Gate Valve Closed?", "Is M123 to OAP gate valve opened?", "Is M123 to OAP gate valve closed?", "Is OAP to BLT gate valve opened?", "Is OAP to BTL Gate Valve Closed?", "Is BLT to TARGET gate valve opened?", "Is BTL to TARGET Gate Valve Closed?", "Is TARGET to BLT2 gate valve opened?", "Is TARGET to BTL2 Gate Valve Closed?", "Is BLT2 to HPD gate valve opened?", "Is BTL2 to HPD Gate Valve Closed?", "Is COMP at Atmospheric Pressure?", "Is M123 at Atmospheric Pressure?", "Is BeamDump at Atmospheric Pressure?", "Is OAP at Atmospheric Pressure?", "Is BLT at Atmospheric Pressure", "Is TARGET at Atmospheric Pressure?", "Is BLT2 at Atmospheric Pressure?", "Is HPD at Atmospheric Pressure?", "Is the EC Roughing Pump ON?", "Is the EC Roughing Pump OFF?", "Does the EC Roughing Pump have a fault?", "Is the LB Roughing Pump ON?", "Is the LB Roughing Pump Off?", "Does the LB Roughing Pump have a fault?", "Is the EC Backing Pump ON?", "Is the EC Backing Pump OFF?", "Is the LB Backing Pump ON?", "Is the LB Backing Pump OFF?", "Does the EC Backing Pump have a fault?", "Does the LB Backing Pump have a fault?", "Is the EC Backing Pipe at Atmospheric Pressure", "Is the LB Backing Pipe at Atmospheric Pressure", "Is the EC Backing Manifold at Atmospheric Pressure", "s the LB Backing Manifold at Atmospheric Pressure?", "Is the EC Roughing Pipe at Atmospheric Pressure", "Is the LB Roughing Pipe at Atmospheric Pressure?", "Is the EC Roughing Manifold at Atmospheric Pressure", "Is the LB Roughing Manifold at Atmospheric Pressure", "Is LB Backing Manifold Valve Opened?", "Is EC Backing Manifold Valve Opened?", "Is LB Roughing Manifold Valve Opened?", "Is EC Roughing Manifold Valve Opened?", "Is COMP Roughing Valve Opened?", "Is M123 Roughing Valve Opened?", "Is M123 Roughing Valve Closed?", "Is OAP Roughing Valve Opened?", "Is OAP Roughing Valve Closed?", "Is HPBD Roughing Valve Opened?", "Is HPBD Roughing Valve Closed?", "Is BTL Roughing Valve Opened?", "Is BTL Roughing Valve Closed?", "Is TARGET Roughing Valve Opened?", "Is TARGET Roughing Valve Closed?", "Is BTL2 Roughing Valve Opened?", "Is BTL2 Roughing Valve Closed?", "Is HPD Roughing Valve Opened?", "Is HPD Roughing Valve Closed?", "Is COMP Turbo Backing Valve Opened?", "Is M123 Turbo Backing Valve Opened", "Is HPBD Turbo Backing Valve Opened?", "Is OAP Turbo Backing Valve Opened?", "Is BTL Turbo Backing Valve Opened?", "Is TARGET1 Turbo Backing Valve Opened?", "Is TARGET2 Turbo Backing Valve Opened?", "Is BTL2 Turbo Backing Valve Opened?", "Is HPD Turbo Backing Valve Opened?", "Is M123 Backing at MID-VAC?", "Is OAP Backing at MID-VAC?", "Is TARGET1 Backing at MID-VAC?", "Is TARGET2 Backing at MID-VAC?", "Is BTL Backing at MID-VAC?", "Is BTL2 Backing at MID-VAC?", "Is HPD Backing at MID-VAC?", "Is M123 Turbo in Normal Operation", "Is COMP Turbo in Normal Operation", "Is OAP Turbo in Normal Operation", "Is BTL Turbo in Normal Operation", "Is TARGET1 Turbo in Normal Operation", "Is TARGET2 Turbo in Normal Operation", "Is BTL2 Turbo in Normal Operation", "Is HPD Turbo in Normal Operation", "Is M123 at MID-VAC?", "Is OAP at MID-VAC?", "Is COMP at MID-VAC?", "Is BTL at MID-VAC?", "Is TARGET at MID-VAC?", "Is BTL2 at MID-VAC?", "Is HPD at MID-VAC?"]
          }
          frame "HPD" {
            w1703 = T32[] [enum."Is HPD Roughing Valve Opened?"] items=["No Action", "Is EC GPM Mode ON?", "Is EC GPM Mode Off?", "Is EC GVM Mode ON?", "Is EC GVM Off?", "Is  EC GPM or GVM Mode ON?", "Is LB GPM Mode ON?", "Is LB GPM Mode Off?", "Is LB GVM Mode ON?", "Is LB GVM Mode Off?", "Is  LB GPM or GVM Mode ON?", "Is M123 Turbo Gate Valve Opened? ", "Is M123 Turbo Gate Valve Closed?", "Is OAP Turbo Gate Valve Opened?", "Is OAP Turbo Gate Valve Closed?", "Is BTLTurbo Gate Valve Opened?", "Is BTL Turbo Gate Valve Closed?", "Is TARGET Turbo Gate Valve 1Opened?", "Is TARGET1 Turbo Gate Valve Closed?", "Is TARGET Turbo Gate Valve 2 Opened?", "Is TAREGT2 Turbo Gate Valve Closed?", "Is BTL2 Turbo Gate Valve Opened?", "Is BTL2 Turbo Gate Valve Closed?", "Is HPD Turbo Gate Valve Opened?", "Is HPD Turbo Gate Valve Closed?", "Is COMP to M123 gate Valve Opened?", "Is COMP to M123 Valve Closed?", "Is HPBD Gate Valve Opened?", "Is HPBD Gate Valve Closed?", "Is M123 to OAP gate valve opened?", "Is M123 to OAP gate valve closed?", "Is OAP to BLT gate valve opened?", "Is OAP to BTL Gate Valve Closed?", "Is BLT to TARGET gate valve opened?", "Is BTL to TARGET Gate Valve Closed?", "Is TARGET to BLT2 gate valve opened?", "Is TARGET to BTL2 Gate Valve Closed?", "Is BLT2 to HPD gate valve opened?", "Is BTL2 to HPD Gate Valve Closed?", "Is COMP at Atmospheric Pressure?", "Is M123 at Atmospheric Pressure?", "Is BeamDump at Atmospheric Pressure?", "Is OAP at Atmospheric Pressure?", "Is BLT at Atmospheric Pressure", "Is TARGET at Atmospheric Pressure?", "Is BLT2 at Atmospheric Pressure?", "Is HPD at Atmospheric Pressure?", "Is the EC Roughing Pump ON?", "Is the EC Roughing Pump OFF?", "Does the EC Roughing Pump have a fault?", "Is the LB Roughing Pump ON?", "Is the LB Roughing Pump Off?", "Does the LB Roughing Pump have a fault?", "Is the EC Backing Pump ON?", "Is the EC Backing Pump OFF?", "Is the LB Backing Pump ON?", "Is the LB Backing Pump OFF?", "Does the EC Backing Pump have a fault?", "Does the LB Backing Pump have a fault?", "Is the EC Backing Pipe at Atmospheric Pressure", "Is the LB Backing Pipe at Atmospheric Pressure", "Is the EC Backing Manifold at Atmospheric Pressure", "s the LB Backing Manifold at Atmospheric Pressure?", "Is the EC Roughing Pipe at Atmospheric Pressure", "Is the LB Roughing Pipe at Atmospheric Pressure?", "Is the EC Roughing Manifold at Atmospheric Pressure", "Is the LB Roughing Manifold at Atmospheric Pressure", "Is LB Backing Manifold Valve Opened?", "Is EC Backing Manifold Valve Opened?", "Is LB Roughing Manifold Valve Opened?", "Is EC Roughing Manifold Valve Opened?", "Is COMP Roughing Valve Opened?", "Is M123 Roughing Valve Opened?", "Is M123 Roughing Valve Closed?", "Is OAP Roughing Valve Opened?", "Is OAP Roughing Valve Closed?", "Is HPBD Roughing Valve Opened?", "Is HPBD Roughing Valve Closed?", "Is BTL Roughing Valve Opened?", "Is BTL Roughing Valve Closed?", "Is TARGET Roughing Valve Opened?", "Is TARGET Roughing Valve Closed?", "Is BTL2 Roughing Valve Opened?", "Is BTL2 Roughing Valve Closed?", "Is HPD Roughing Valve Opened?", "Is HPD Roughing Valve Closed?", "Is COMP Turbo Backing Valve Opened?", "Is M123 Turbo Backing Valve Opened", "Is HPBD Turbo Backing Valve Opened?", "Is OAP Turbo Backing Valve Opened?", "Is BTL Turbo Backing Valve Opened?", "Is TARGET1 Turbo Backing Valve Opened?", "Is TARGET2 Turbo Backing Valve Opened?", "Is BTL2 Turbo Backing Valve Opened?", "Is HPD Turbo Backing Valve Opened?", "Is M123 Backing at MID-VAC?", "Is OAP Backing at MID-VAC?", "Is TARGET1 Backing at MID-VAC?", "Is TARGET2 Backing at MID-VAC?", "Is BTL Backing at MID-VAC?", "Is BTL2 Backing at MID-VAC?", "Is HPD Backing at MID-VAC?", "Is M123 Turbo in Normal Operation", "Is COMP Turbo in Normal Operation", "Is OAP Turbo in Normal Operation", "Is BTL Turbo in Normal Operation", "Is TARGET1 Turbo in Normal Operation", "Is TARGET2 Turbo in Normal Operation", "Is BTL2 Turbo in Normal Operation", "Is HPD Turbo in Normal Operation", "Is M123 at MID-VAC?", "Is OAP at MID-VAC?", "Is COMP at MID-VAC?", "Is BTL at MID-VAC?", "Is TARGET at MID-VAC?", "Is BTL2 at MID-VAC?", "Is HPD at MID-VAC?"]
          }
        }
        n647 = call "GetAction.vi"("Check Condition"=w1678, "Query Array"=w1674, "input cluster"=w1667, "error in (no error)"=w1680) -> ("Status Array Out"=w1679:string[], "Generate Event?"=w1664:bool, "error out"=w1676:errorcluster)  [unwired: 6 in, 3 out]
